vi "Test Serializer.Text.vi"(8 "error in (no error)":errorcluster) -> (0 "error out":errorcluster)   [LabVIEW 2013]
uses:
  source/Serializer.PlainText/Serializer.PlainText.lvclass
  <vilib>/addons/_JKI Toolkits/Caraya/classes/Assert/Assert Equal Value and Type_Variant.vi
  <vilib>/addons/_JKI Toolkits/Caraya/classes/Assert/Assert Equal Value_Variant.vi
  <vilib>/addons/_JKI Toolkits/Caraya/classes/Assert/Assert Not Error.vi
  <vilib>/addons/_JKI Toolkits/Caraya/classes/Assert/Assert Almost Equal_Float.vi
  <vilib>/addons/_JKI Toolkits/Caraya/classes/Assert/Assert.lvclass
  source/Serializer/Serializer.lvclass
  <vilib>/addons/_JKI Toolkits/Caraya/classes/Test/Test.lvclass
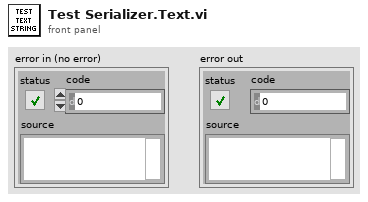
[diagram p1: front panel]
types:
  T1 = cluster{"error":errorcluster, "EnumU16":enum16{"A", "B", "C"}, "Value":dbl}
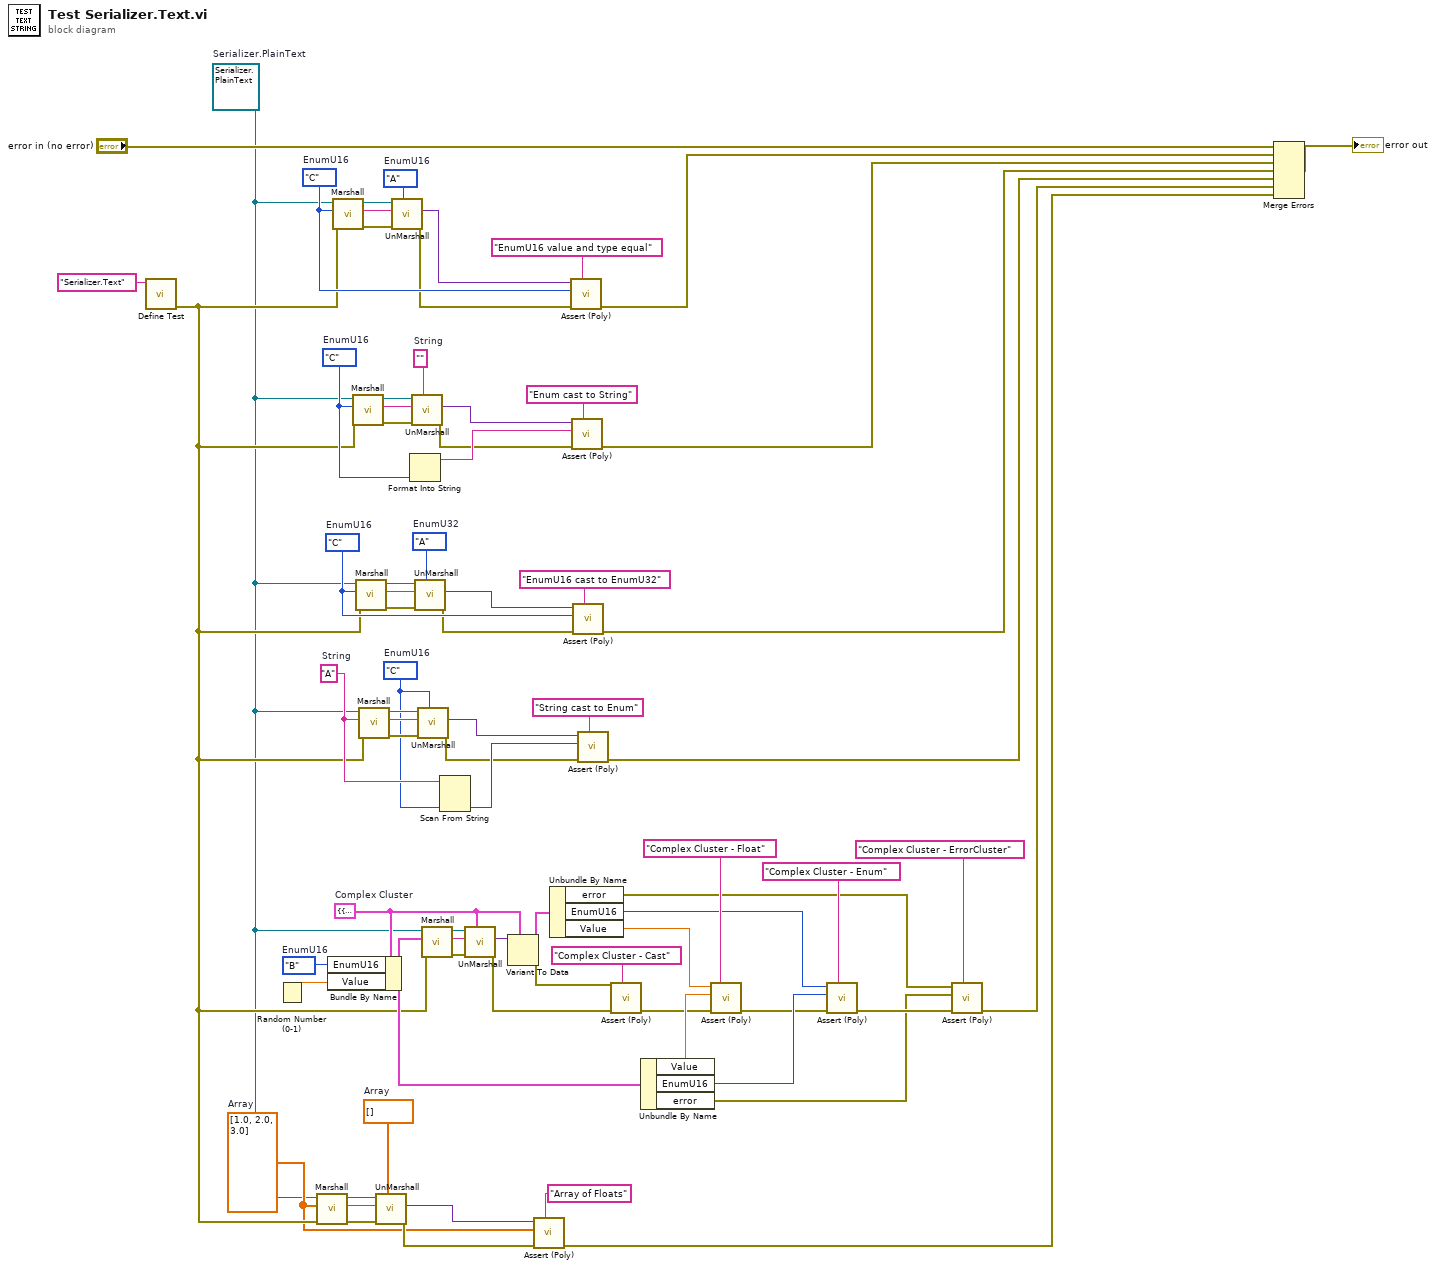
[diagram p0: block diagram]
diagram:
  w1 = refnum<class "Serializer.PlainText.lvclass"> refnum  # Serializer.PlainText
  w3 = dbl[] [1.0, 2.0, 3.0]  # Array
  w4 = dbl[] []  # Array
  w38 = enum16{"A", "B", "C"}."B"  # EnumU16
  w28 = T1 {"error"={"status"=FALSE, "code"=0, "source"=""}, "EnumU16"=enum."A", "Value"=0.0}  # Complex Cluster
  w44 = "A"  # String
  w43 = enum16{"A", "B", "C"}."C"  # EnumU16
  w56 = enum32{"A", "B", "C"}."A"  # EnumU32
  w51 = enum16{"A", "B", "C"}."C"  # EnumU16
  w65 = ""  # String
  w54 = enum16{"A", "B", "C"}."C"  # EnumU16
  w74 = enum16{"A", "B", "C"}."A"  # EnumU16
  w76 = enum16{"A", "B", "C"}."C"  # EnumU16
  n1 = call <vilib>:"Define Test.vi"("Label (VI Title)"="Serializer.Text") -> ("error out"=w5:errorcluster)  [unwired: 10 in]
  n2 = Random Number (0-1)() -> (number: 0 to 1=w37:dbl)
  n3 = call "Marshall.vi"("error in (no error)"=w5, "Variant"=w3, "Serializer in"=w1) -> ("error out"=w6:errorcluster, "String"=w8:string, "Serializer out"=w9:refnum<class "Serializer.PlainText.lvclass">)  [unwired: 6 in]
  n4 = Bundle By Name(cluster=w28, "EnumU16"=w38, "Value"=w37) -> (w24:T1)
  n5 = call "Marshall.vi"("error in (no error)"=w5, "Variant"=w76, "Serializer in"=w1) -> ("error out"=w33:errorcluster, "String"=w73:string, "Serializer out"=w72:refnum<class "Serializer.PlainText.lvclass">)  [unwired: 6 in]
  n6 = call "Marshall.vi"("error in (no error)"=w5, "Variant"=w54, "Serializer in"=w1) -> ("error out"=w62:errorcluster, "String"=w66:string, "Serializer out"=w67:refnum<class "Serializer.PlainText.lvclass">)  [unwired: 6 in]
  n7 = call "Marshall.vi"("error in (no error)"=w5, "Variant"=w51, "Serializer in"=w1) -> ("error out"=w61:errorcluster, "String"=w59:string, "Serializer out"=w58:refnum<class "Serializer.PlainText.lvclass">)  [unwired: 6 in]
  n8 = call "Marshall.vi"("error in (no error)"=w5, "Variant"=w44, "Serializer in"=w1) -> ("error out"=w49:errorcluster, "String"=w47:string, "Serializer out"=w46:refnum<class "Serializer.PlainText.lvclass">)  [unwired: 6 in]
  n9 = call "UnMarshall.vi"("Type"=w4, "error in (no error)"=w6, "String"=w8, "Serializer in"=w9) -> ("error out"=w11:errorcluster, "Variant"=w10:variant)  [unwired: 5 in, 1 out]
  n10 = call "UnMarshall.vi"("Type"=w74, "error in (no error)"=w33, "String"=w73, "Serializer in"=w72) -> ("error out"=w32:errorcluster, "Variant"=w75:variant)  [unwired: 5 in, 1 out]
  n11 = Format Into String(w54) -> (resulting string=w53:string)  [unwired: 3 in, 1 out]
  n12 = call "UnMarshall.vi"("Type"=w65, "error in (no error)"=w62, "String"=w66, "Serializer in"=w67) -> ("error out"=w34:errorcluster, "Variant"=w55:variant)  [unwired: 5 in, 1 out]
  n13 = call "UnMarshall.vi"("Type"=w56, "error in (no error)"=w61, "String"=w59, "Serializer in"=w58) -> ("error out"=w35:errorcluster, "Variant"=w52:variant)  [unwired: 5 in, 1 out]
  n14 = call "UnMarshall.vi"("Type"=w43, "error in (no error)"=w49, "String"=w47, "Serializer in"=w46) -> ("error out"=w36:errorcluster, "Variant"=w50:variant)  [unwired: 5 in, 1 out]
  n15 = call "Marshall.vi"("error in (no error)"=w5, "Variant"=w24, "Serializer in"=w1) -> ("error out"=w31:errorcluster, "String"=w40:string, "Serializer out"=w41:refnum<class "Serializer.PlainText.lvclass">)  [unwired: 6 in]
  n16 = Scan From String(input string=w44, default 1=w43) -> (output 1=w42:enum16{"A", "B", "C"})  [unwired: 3 in, 3 out]
  n17 = call "UnMarshall.vi"("Type"=w28, "error in (no error)"=w31, "String"=w40, "Serializer in"=w41) -> ("error out"=w30:errorcluster, "Variant"=w29:variant)  [unwired: 5 in, 1 out]
  n18 = Variant To Data(type=w28, Variant=w29) -> (data=w26:T1, error out=w27:errorcluster)  [unwired: 1 in]
  n19 = call-poly <vilib>:"Assert (Poly).vi"("Label"="Array of Floats", "error in (no error)"=w11, "Y"=w3, "X"=w10) -> ("error out"=w2:errorcluster)  [unwired: 7 in]
  n20 = Unbundle By Name(w26) -> ("error"=w13:errorcluster, "EnumU16"=w20:enum16{"A", "B", "C"}, "Value"=w25:dbl)
  n21 = call-poly <vilib>:"Assert (Poly).vi"("Label"="EnumU16 value and type equal", "error in (no error)"=w32, "Y"=w76, "X"=w75) -> ("error out"=w68:errorcluster)  [unwired: 7 in]
  n22 = call-poly <vilib>:"Assert (Poly).vi"("Label"="Enum cast to String", "error in (no error)"=w34, "Y"=w53, "X"=w55) -> ("error out"=w63:errorcluster)  [unwired: 7 in]
  n23 = call-poly <vilib>:"Assert (Poly).vi"("Label"="EnumU16 cast to EnumU32", "error in (no error)"=w35, "Y"=w51, "X"=w52) -> ("error out"=w57:errorcluster)  [unwired: 7 in]
  n24 = call-poly <vilib>:"Assert (Poly).vi"("Label"="String cast to Enum", "error in (no error)"=w36, "Y"=w42, "X"=w50) -> ("error out"=w45:errorcluster)  [unwired: 7 in]
  n25 = call-poly <vilib>:"Assert (Poly).vi"("Label"="Complex Cluster - Cast", "error in (no error)"=w30, "Not Error?"=w27) -> ("error out"=w22:errorcluster)  [unwired: 8 in]
  n26 = Unbundle By Name(w24) -> ("Value"=w23:dbl, "EnumU16"=w18:enum16{"A", "B", "C"}, "error"=w12:errorcluster)
  n27 = call-poly <vilib>:"Assert (Poly).vi"("Label"="Complex Cluster - Float", "error in (no error)"=w22, "Y"=w23, "X"=w25) -> ("error out"=w17:errorcluster)  [unwired: 7 in]
  n28 = call-poly <vilib>:"Assert (Poly).vi"("Label"="Complex Cluster - Enum", "error in (no error)"=w17, "Y"=w18, "X"=w20) -> ("error out"=w16:errorcluster)  [unwired: 7 in]
  n29 = call-poly <vilib>:"Assert (Poly).vi"("Label"="Complex Cluster - ErrorCluster", "error in (no error)"=w16, "Y"=w12, "X"=w13) -> ("error out"=w15:errorcluster)  [unwired: 7 in]
  n30 = Merge Errors("error in (no error)", w68, w63, w57, w45, w15, w2) -> (→"error out":errorcluster)
